vi "Restore original Coordinates.vi"(6 "temp size in":T1={"left"=0, "top"=0, "right"=32, "bottom"=32}, 11 "Pic in":picture) -> (3 "Pic out":picture)   [LabVIEW 2020, in "lv_icon.lvlib"]
doc: "Restore the original coordinates after messing with the Image Data."
uses:
  lv_icon.lvlib
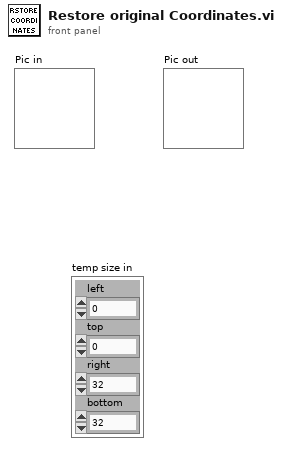
[diagram p1: front panel]
types:
  T1 = cluster{"left":i16, "top":i16, "right":i16, "bottom":i16}
  T2 = typedef "imagedata.ctl" = cluster{"image type":i32, "image depth":i32, "image":u8[], "mask":u8[], "colors":u32[], "Rectangle":cluster{"left":i16, "top":i16, "right":i16, "bottom":i16}}
  T3 = cluster{"left":i16, "top":i16, "left":i16, "top":i16}
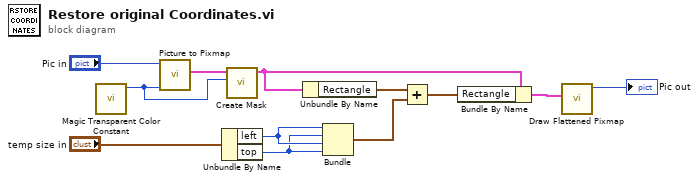
[diagram p0: block diagram]
diagram:
  n1 = call "Magic Transparent Color Constant.vi"() -> ("Magic transparent color constant"=w10:u32)  [unwired: 11 out]
  n2 = call <vilib>:"Picture to Pixmap.vi"("Background Color"=w10, "picture"="Pic in") -> ("image data"=w11:T2)  [unwired: 2 in, 7 out]
  n3 = Unbundle By Name("temp size in") -> ("left"=w2:i16, "top"=w1:i16)
  n4 = call <vilib>:"Create Mask.vi"("Mask Color (Black)"=w10, "image data"=w11) -> ("image data"=w7:T2)  [unwired: 2 in, 7 out]
  n5 = Unbundle By Name(w7) -> ("Rectangle"=w9:T1)
  n6 = Bundle("left"=w2, "top"=w1, "left"=w2, "top"=w1) -> (w5:T3)  [unwired: 1 out]
  n7 = Add(x=w9, y=w5) -> (x+y=w8:cluster{"left":i16, "top":i16, i16, i16})
  n8 = Bundle By Name(cluster=w7, "Rectangle"=w8) -> (w6:T2)
  n9 = call <vilib>:"Draw Flattened Pixmap.vi"("image data"=w6) -> ("new picture"=→"Pic out":picture)  [unwired: 1 in, 7 out]
